vi "Simple DataSocket - Reader.vi"() -> ()   [LabVIEW 2019]
doc: "Uses DataSocket to read array data. \n \nThe Writer, Server, and Reader can all be on the same computer or different computers. The Writer and Reader URLs should point to the computer where the DataSocket Server is."
panel:
  in  "Stop":bool
  out "Data Read":dbl[](graph)
  # "Overview: Demonstrates the use of the DataSocket functions to read data from the DataSocket server.\nRequirements: Windows\nInstructions:\n1. Ensure Simple DataSocket - Writer.vi is already running.\n2. Run the VI.\n3. Click Stop to stop the VI."
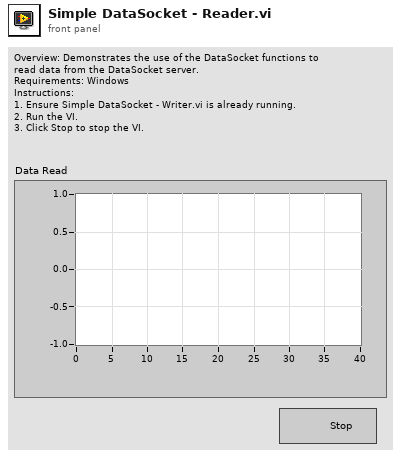
[diagram p1: front panel]
types:
  T1 = enum16{"Read", "Write", "ReadWrite", "BufferedRead", "BufferedReadWrite"}
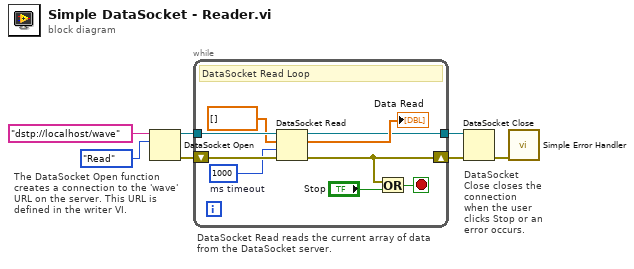
[diagram p0: block diagram]
diagram:
  # "The DataSocket Open function creates a connection to the 'wave' URL on the server. This URL is defined in the writer VI."
  # "DataSocket Read reads the current array of data from the DataSocket server."
  # "DataSocket Close closes the connection when the user clicks Stop or an error occurs."
  n1 = DataSocket Open(10:T1."Read" ("mode"), 11:"dstp://localhost/wave" ("Read Location")) -> (0:w5:errorcluster, 3:w6:refnum<k13>)  [unwired: 2 in]
  n2 = while {
    tunnel: w6 -> [w14]
    tunnel: [w9] -> w1
    shift-right: [w10] -> w4
    shift-left: w5 -> [w12]
    stop <- w15 stop-if-true
    w11 = 1000  # ms timeout
    # "DataSocket Read Loop"
    n3 = DataSocket Read(8:w12, 9:w11, 10:dbl[] [], 11:w14) -> (0:w10:errorcluster, 2:→"Data Read":dbl[], 3:w9:refnum<k13>)  [unwired: 5 out]
    n4 = Or(x=w10, y="Stop") -> (x .or. y?=w15:bool)
  }
  n5 = DataSocket Close(8:w4, 11:w1) -> (0:w2:errorcluster)  [unwired: 1 in, 1 out]
  n6 = call <vilib>:"Simple Error Handler.vi"("error in (no error)"=w2) -> ()  [unwired: 4 in, 5 out]
